vi "Configure Averaging.vi"(7 "Enable THD Sync Averaging (T: Enable)":bool=TRUE, 8 "error in (no error)":errorcluster, 9 "THD Averaging (0: avgFast)":i32(ring) items=["avgFast", "avgOnedB", "avgHalfdB", "avgTenthdB"], 10 "Analyzer (0: A0)":i32(ring) items=["A0", "A1"], 11 "VISA resource name":refnum<visa-resource-name>) -> (0 "error out":errorcluster, 3 "VISA resource name out":refnum<visa-resource-name>)   [LabVIEW 2014, in "Stanford Research SR1.lvlib"]
doc: "Configures the attributes of the THD Averaging."
uses:
  Stanford Research SR1.lvlib
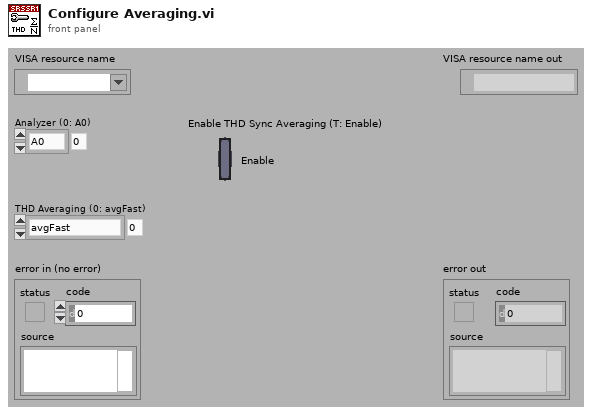
[diagram p1: front panel]
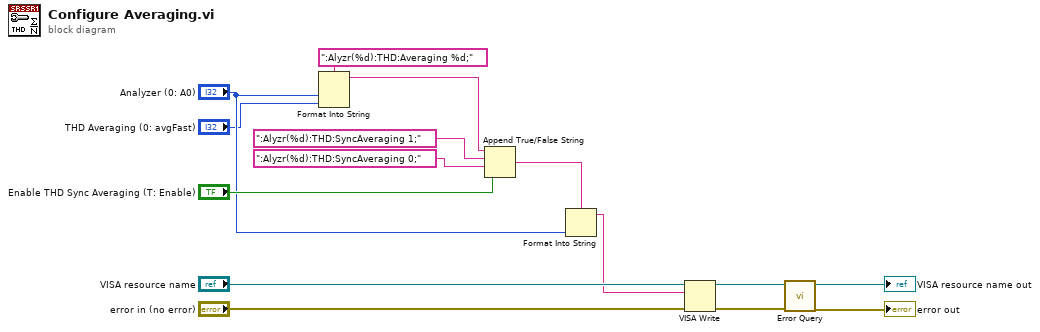
[diagram p0: block diagram]
diagram:
  n1 = Format Into String(format string=":Alyzr(%d):THD:Averaging %d;", "Analyzer (0: A0)", "THD Averaging (0: avgFast)") -> (resulting string=w14:string)  [unwired: 2 in, 1 out]
  n2 = Append True/False String(1:"Enable THD Sync Averaging (T: Enable)", 2:":Alyzr(%d):THD:SyncAveraging 0;", 3:":Alyzr(%d):THD:SyncAveraging 1;", 4:w14) -> (0:w4:string)
  n3 = Format Into String(format string=w4, "Analyzer (0: A0)") -> (resulting string=w1:string)  [unwired: 2 in, 1 out]
  n4 = VISA Write(VISA resource name="VISA resource name", write buffer=w1, error in (no error)="error in (no error)") -> (VISA resource name out=w8:refnum<visa-resource-name>, error out=w7:errorcluster)  [unwired: 1 out]
  n5 = call "Error Query.vi"("error in (no error)"=w7, "VISA resource name"=w8) -> ("error out"=→"error out":errorcluster, "VISA resource name out"=→"VISA resource name out":refnum<visa-resource-name>)  [unwired: 6 in, 2 out]
